vi "initial key.vi"(10 "clé initiale":u8[][](array[numeric])) -> (1 "Z0":dbl format="%#_15g", 2 "Y0":dbl format="%#_14g", 3 "X0":dbl)   [LabVIEW 2019]
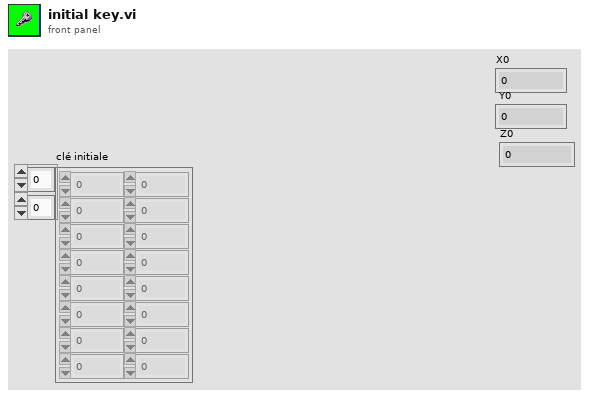
[diagram p1: front panel]
types:
  T1 = cluster{"clé initiale [0]":u8, "clé initiale [1]":u8, "clé initiale [2]":u8, "clé initiale [3]":u8, "clé initiale [4]":u8, "clé initiale [5]":u8, "clé initiale [6]":u8, "clé initiale [7]":u8, "clé initiale [8]":u8}
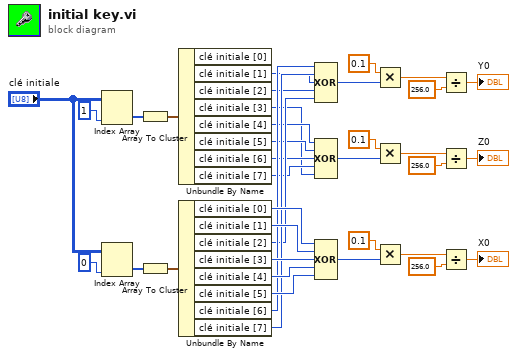
[diagram p0: block diagram]
diagram:
  n1 = Index Array(array="clé initiale", index (col)=1) -> (element=w17:u8[])  [unwired: 1 in]
  n2 = Index Array(array="clé initiale", index (col)=0 ("disabled index (col)")) -> (element=w20:u8[])  [unwired: 1 in]
  n3 = Array To Cluster(array=w17) -> (cluster=w16:T1)
  n4 = Array To Cluster(array=w20) -> (cluster=w22:T1)
  n5 = Unbundle By Name(w16) -> ("clé initiale [1]"=w7:u8, "clé initiale [2]"=w6:u8, "clé initiale [3]"=w1:u8, "clé initiale [4]"=w5:u8, "clé initiale [5]"=w4:u8, "clé initiale [6]"=w3:u8, "clé initiale [7]"=w2:u8)  [unwired: 1 out]
  n6 = Unbundle By Name(w22) -> ("clé initiale [0]"=w15:u8, "clé initiale [1]"=w14:u8, "clé initiale [2]"=w8:u8, "clé initiale [3]"=w13:u8, "clé initiale [4]"=w12:u8, "clé initiale [5]"=w11:u8, "clé initiale [6]"=w10:u8, "clé initiale [7]"=w9:u8)
  n7 = Compound Arithmetic op=XOR(w10, w9, w7, w6, w8) -> (w27:u8)
  n8 = Compound Arithmetic op=XOR(w5, w4, w3, w2, w1) -> (w26:u8)
  n9 = Compound Arithmetic op=XOR(w15, w14, w13, w12, w11) -> (w36:u8)
  n10 = Multiply(x=0.1, y=w27) -> (x*y=w32:dbl)
  n11 = Multiply(x=0.1, y=w26) -> (x*y=w29:dbl)
  n12 = Multiply(x=0.1, y=w36) -> (x*y=w35:dbl)
  n13 = Divide(x=w32, y=256.0) -> (x/y=→"Y0":dbl)
  n14 = Divide(x=w29, y=256.0) -> (x/y=→"Z0":dbl)
  n15 = Divide(x=w35, y=256.0) -> (x/y=→"X0":dbl)
